vi "play_FXP_AFMss_MPC_DistEst_singleAxisN22.vi"() -> ()   [LabVIEW 2017]
uses:
  fpga_VIs/fixed-point/single-axis/fxp_mpc/fgm_pipiline/quadProgParams_pipe.ctl
  fpga_VIs/fixed-point/typeDefs/FXPControlParams_distEst.ctl
  <vilib>/Analysis/Matrix/Datatypes/RealMatrix.ctl
  fpga_fp_interface_lib/fpga_interface_types/boolean_indicators.ctl
  controls/ObserverMatrices.ctl
  <vilib>/userdefined/High Color/nirio_resource_hc.ctl
  <vilib>/Utility/error.llb/DialogType.ctl
  <vilib>/Utility/file.llb/Read Delimited Spreadsheet (DBL).vi
  <vilib>/FPGAPlugInAG/cRIO-9082/niLvFpga_Open_cRIO-9082.vi
  <vilib>/rvi/interface/common/dynamic/niFpgaDynamicAddResources.vi
  <vilib>/FPGAPlugInAG/Dynamic/niLvFpga_Reset_Dynamic.vi
  <vilib>/rvi/interface/common/niFpgaWaitOnOcc.vi
  <vilib>/Utility/error.llb/Error Cluster From Error Code.vi
  <vilib>/rvi/errors/niLvFpgaAdjustHostInterfaceError.vi
  <vilib>/FPGAPlugInAG/Dynamic/niLvFpga_Run_Dynamic.vi
  <vilib>/RVI Host/nirviSupport.llb/nirviErrorClusterFromErrorCode.vi
  fpga_fp_interface_lib/write_FP_data_to_fpga.vi
  fpga_fp_interface_lib/acquire_FXP_18-5_FIFO_1.vi
  <vilib>/Analysis/Matrix/Numeric/Conversions/Array To Matrix - RA2.vi
  <vilib>/Utility/file.llb/Write To Spreadsheet File (DBL).vi
  <vilib>/FPGAPlugInAG/Dynamic/niLvFpga_Close_Dynamic.vi
  <vilib>/rvi/interface/nirviOpenFPGA/nirviOpenFPGA.xnode
  FPGA Bitfiles/XYpeizocontrol_FPGATargetSPARTA_FXP_AFMss_MPC_singleAxis_N22.lvbitx
  <vilib>/rvi/interface/nirviMethod/nirviMethod.xnode
  <vilib>/rvi/interface/nirviReadWriteControl/nirviReadWriteControl.xnode
  <vilib>/rvi/interface/nirviCloseFPGA/nirviCloseFPGA.xnode
  <vilib>/rvi/errors/niLvFpgaMergeErrorWithErrorCode.vi
  <vilib>/rvi/interface/Simulation/niFpgaSimulationCallBeginRW.vi
  <vilib>/rvi/interface/nirviMethod/StockFPGA_InlinedMethodWaitForSingleIRQ.vi
  <vilib>/FPGAPlugInAG/Dynamic/niLvFpga_WaitOnIrq_Dynamic.vi
  <vilib>/FPGAPlugInAG/Dynamic/niLvFpga_AcknowledgeIrq_Dynamic.vi
  <vilib>/FPGAPlugInAG/Dynamic/niLvFpga_ConfigureFifo_Dynamic.vi
  NiFpgaLv.dll
  <vilib>/Analysis/Matrix/NI_Matrix.lvlib
  <vilib>/FPGAPlugInAG/Dynamic/niLvFpga_WriteFifo_Dynamic.vi
  labview/utils_lib/utils.lvlib
panel:
  out "size(s) 4":i32
  out "error out":errorcluster
  out "size(s) 3":i32
  out "size(s) 2":i32
  in  "N_sat":i32
  in  "sat_ws":T1
  in  "sat_ds":T1
  out "Actual Depth":u32
  out "first row":dbl[](array[numeric])
  out "elements left":i32=1
  in  "N_hyst":i32
  in  "w_s":T1
  in  "r_s":T1
  in  "TF Order":i32
  in  "den":T1
  in  "num":T1
  out "u_k out":fxp<+/-,32,5>
  out "size(s)":i32[](array[numeric])
  in  "Tab Control":T2(tab)
  in  "traj_path":path=path "Z:/mpc-journal/step-exps/traj_data.csvtraj_data.csv"
  in  "control_data_path":path=path "Z:/mpc-journal/step-exps/MPCControls01.csv"
  in  "outputDataPath":path=path "Z:/mpc-journal/step-exps/expOut_multiAxis_mpc_tmp.csv"
  in  "dry_run":bool
  out "XY Graph":cluster{dbl[], "2D Data Out":dbl[]}[](graph)
  out "QP_params":T3={"maxIter"=0, "nuN"=24, "Ns_mpc"=0, "-beta"=-0.9987945556640625, "beta+1"=1.9987945556640625}
  out "ControlParams":T4={"umax"=3.0, "Ns_obs/cntrl"=0, "ref_f_VEC"=[0.0, 0.0], "du_max"=0.0}
  in  "TsTicks":i32=1600
  in  "umax":dbl=1.0 format="%#_13g"
  in  "ymax":dbl=4.0 format="%#_13g"
  in  "Iters":i32=25
  in  "SettleTicks":i32=10
  in  "ABORT":bool
  out "Fifo matrix TimeOUt":bool
  in  "ref":dbl=1.0 format="%#_13g"
  out "Loop Ticks (benchmark)":i16
  in  "maxIter":u16=22
  in  "du_max":dbl=1.0 format="%#_13g"
  out "boolean  indicators":T5
  out "error out (stage 2)":errorcluster
  out "Error Out (stage 1)":errorcluster
  out "x-x(0)":fxp<+/-,18,5>
  out "ControlMatrices":T6
  out "MPC matrices":dbl[][](array[numeric])
  out "result_data":T1
  out "Empty Elements Remaining":u32
  # "NOTE: Ns is the number of states in the plant. The number of states in the \nobserver is Ns+1. Thus, for B, L, C, and A, we use NS+1. For K and Xss, we use Ns\nbecause the controller does not operate on the disturbance state, Xd."
  # "yk\nulin\ndu\nu_inv\nIpow\nX"
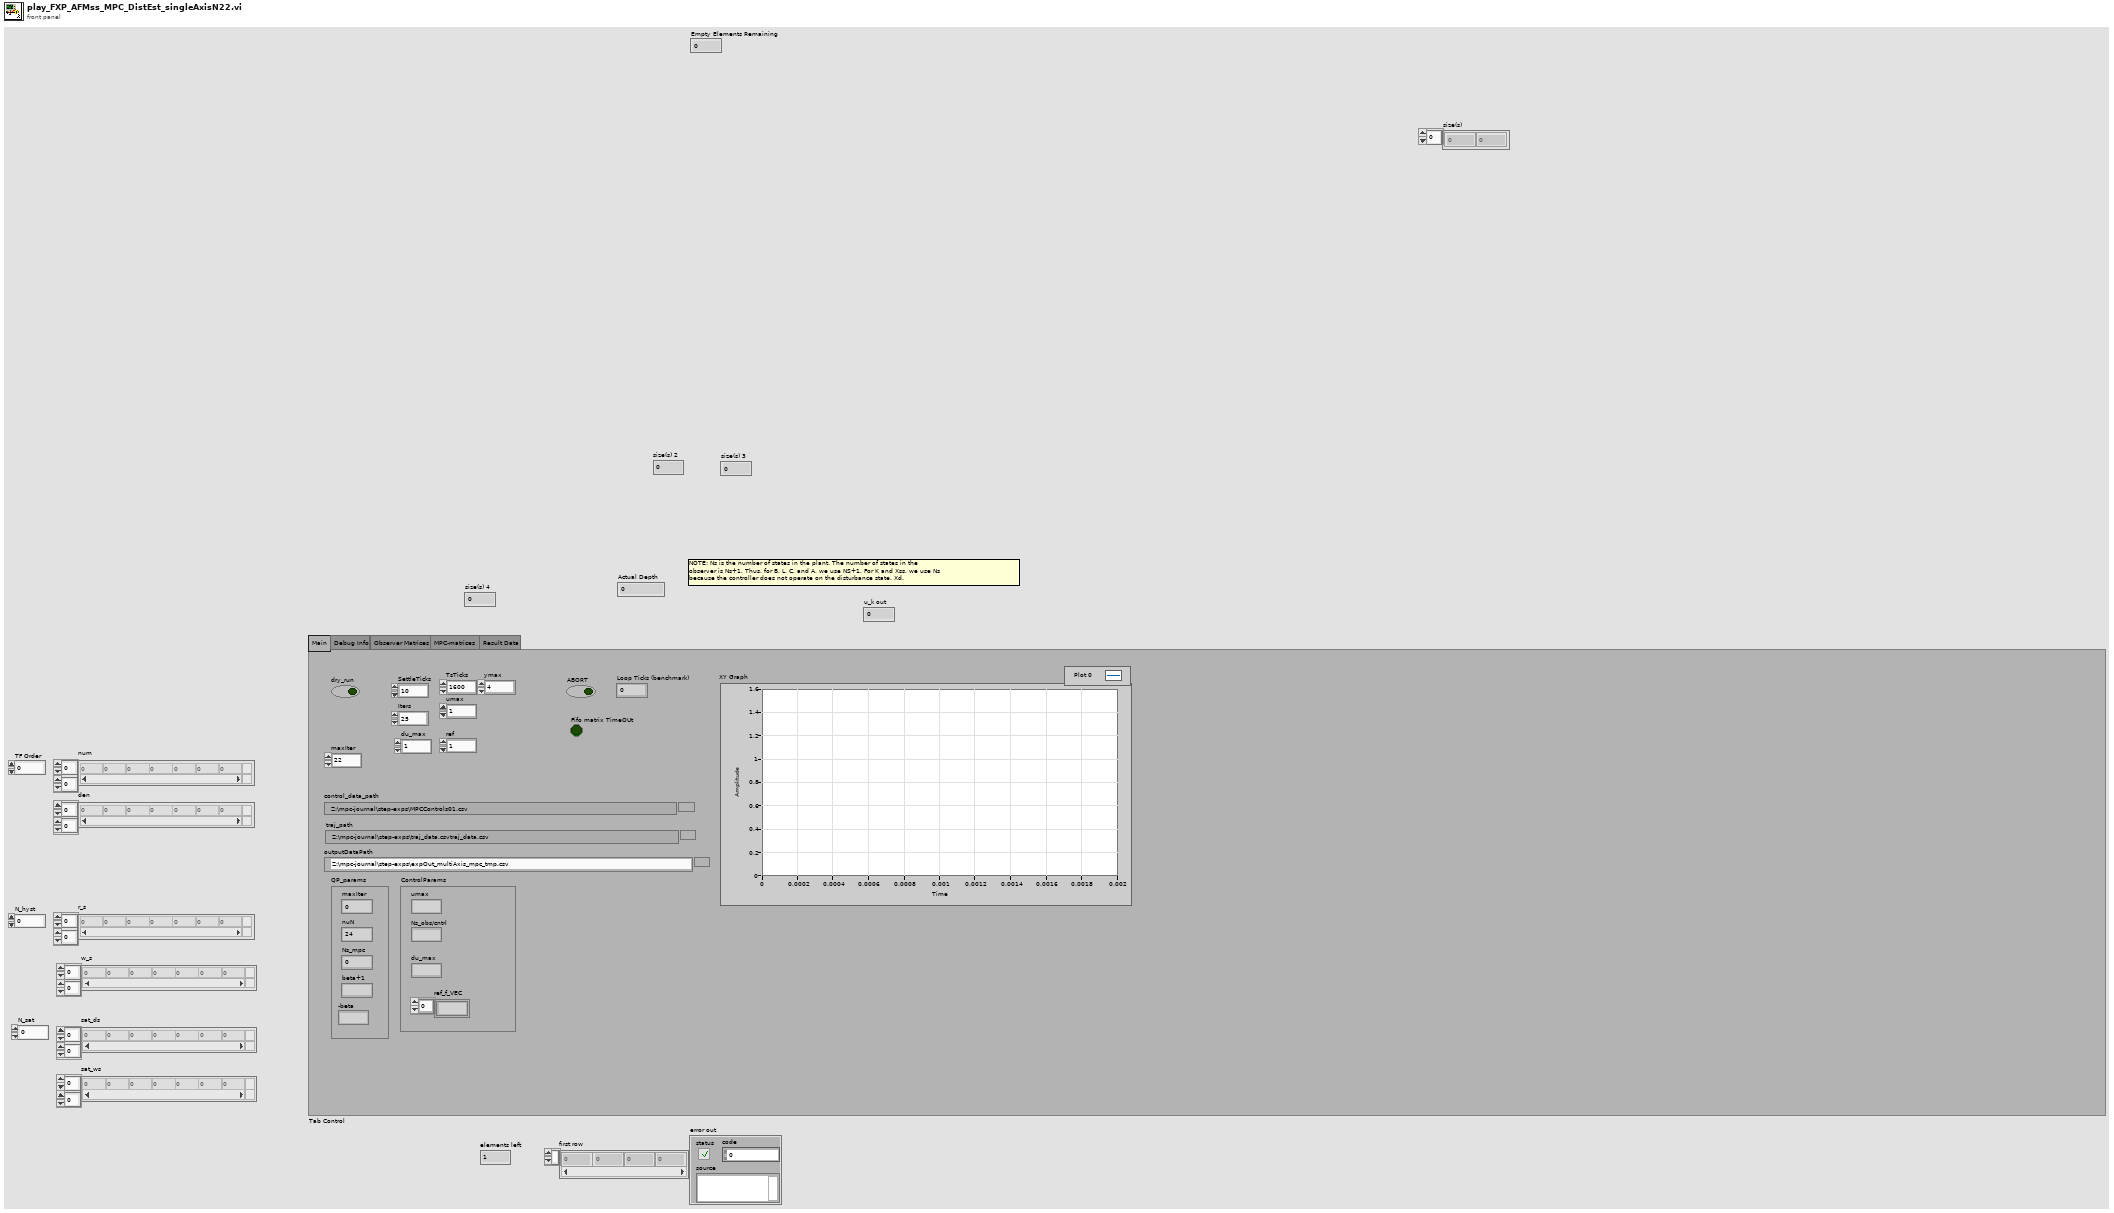
[diagram p1: front panel]
types:
  T1 = typedef "NI_Matrix.lvlib/RealMatrix.ctl" = dbl[][]
  T2 = enum32{"Main", "Debug Info", "Observer Matrices", "MPC-matrices", "Result Data"}
  T3 = typedef "quadProgParams_pipe.ctl" = cluster{"maxIter":u16, "nuN":u16, "Ns_mpc":u16, "-beta":fxp<+/-,18,2>, "beta+1":fxp<+/-,18,2>}
  T4 = typedef "FXPControlParams_distEst.ctl" = cluster{"umax":fxp<+/-,18,5>, "Ns_obs/cntrl":u8, "ref_f_VEC":fxp<+/-,32,5>[], "du_max":fxp<+/-,18,5>}
  T5 = typedef "boolean_indicators.ctl" = cluster{"unstable-z-traj":bool, "input fifo time-out":bool, "logging fifo timeout":bool, "scanning finished":bool, "unstable-x-traj":bool, "unstable-y-traj":bool, "ABORT":bool, "All Measurements Done":bool, "fpga_finished":bool}
  T6 = typedef "ObserverMatrices.ctl" = cluster{"Az":fxp<+/-,32,4>[][], "Bz":dbl[][], "Lz":dbl[][], "Kz":dbl[][], "NxNu":dbl[][]}
  T7 = typedef "nirio_resource_hc.ctl" = tag
  T8 = cluster{"unstable-z-traj":bool, "input fifo time-out":bool, "logging fifo timeout":bool, "scanning finished":bool, "unstable-x-traj":bool, "unstable-y-traj":bool, "ABORT":bool, "All Measurements Done":bool, "fpga_finished":bool}
  T9 = typedef "DialogType.ctl" = u16
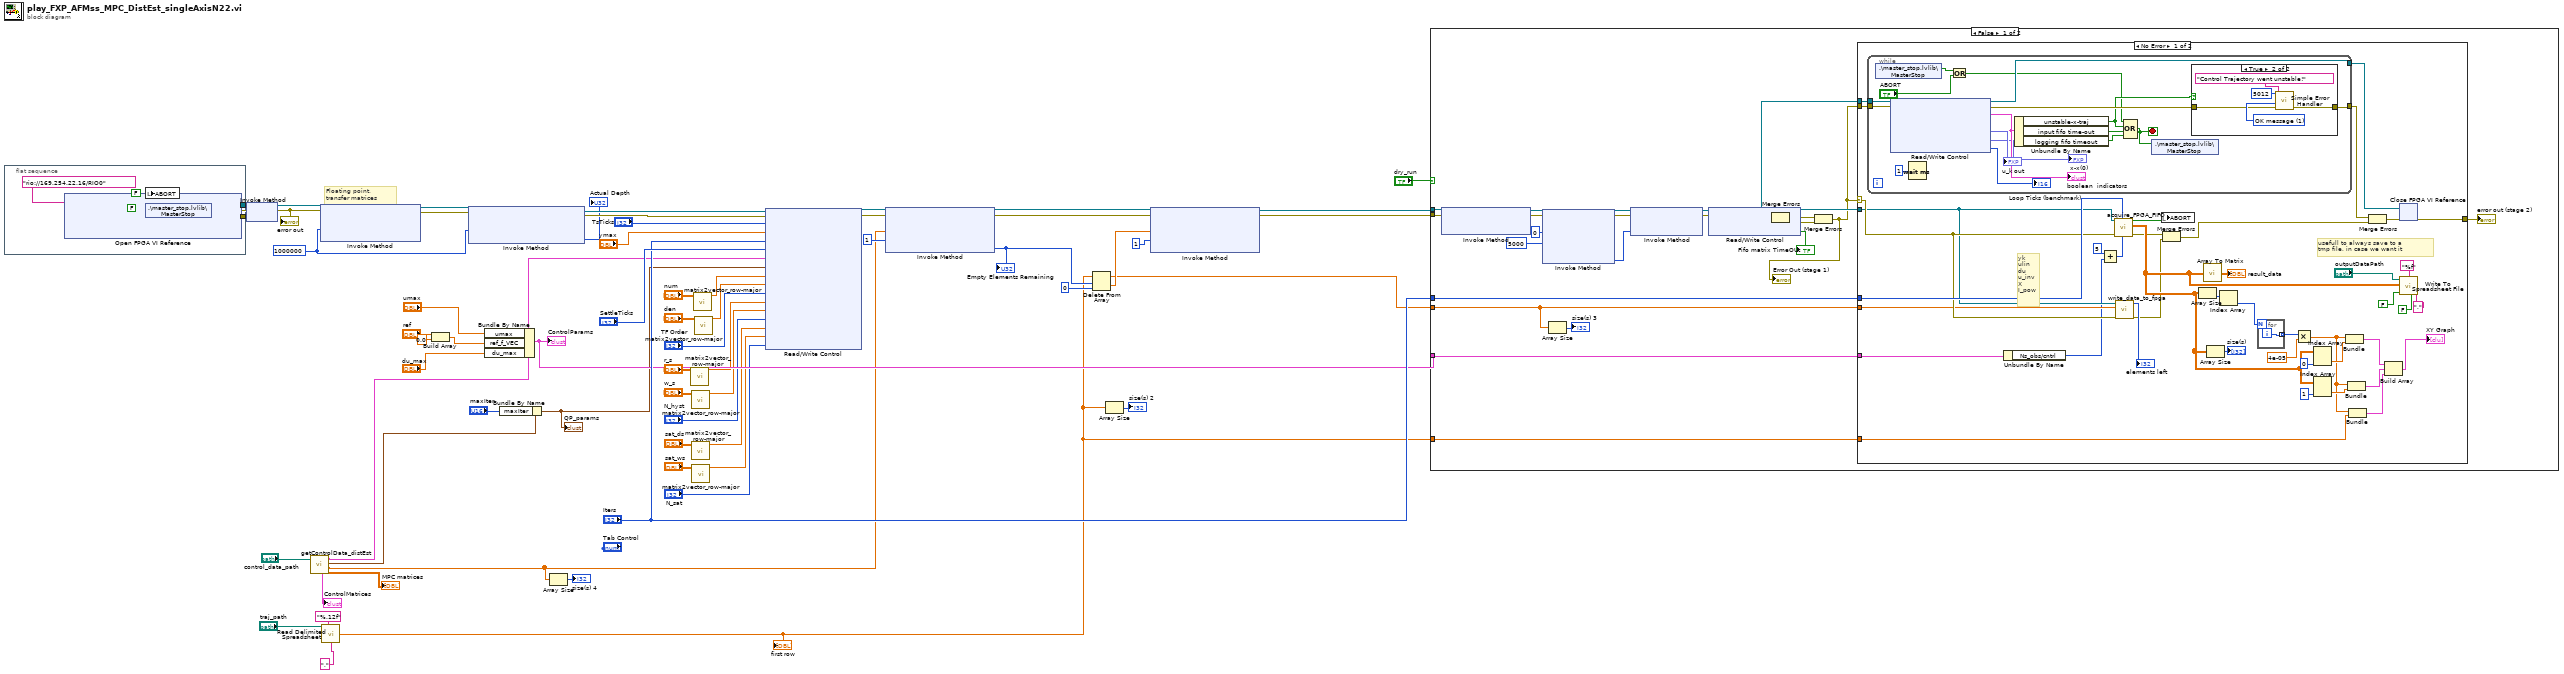
[diagram p0: block diagram]
diagram:
  w43 = u32 1000000 ("Requested Depth")
  # "Floating point, \ntransfer matrices"
  n1 = flat-sequence {
    tunnel: [w65] -> w56
    tunnel: [w67] -> w54
    frame #0 {
      n2 = xnode "Open FPGA VI Reference"("resource name"=T7 "rio://169.254.22.16/RIO0") -> ("FPGA VI Reference Out"=w67:refnum<k20>, "error out"=w64:errorcluster)  [unwired: 1 in]
      n3 = shared-variable ".\\master_stop.lvlib\\MasterStop"(FALSE ("MasterStop"), error in=w64) -> (error out=w65:errorcluster)
      n4 = local write "ABORT"(FALSE ("ABORT")) -> ()
    }
  }
  n5 = xnode "Invoke Method"("FPGA VI Reference In"=w54, "error in"=w56) -> ("FPGA VI Reference Out"=w53:refnum<k20>, "error out"=w52:errorcluster)
  "error out" <- w52
  n6 = call "getControlData_distEst.vi"("system matricec path"="control_data_path") -> ("MPC matrices"=→"MPC matrices":dbl[][], "AllMatrix"=w2:dbl[], "QP_params"=w36:T3, "ControlParams"=w41:T4, "ControlMatrices"=→"ControlMatrices":T6)  [unwired: 6 in]
  n7 = xnode "Invoke Method"("FPGA VI Reference In"=w53, "error in"=w52, "Requested Depth"=w43) -> ("FPGA VI Reference Out"=w51:refnum<k20>, "error out"=w50:errorcluster)  [unwired: 1 out]
  n8 = call-poly <vilib>:"Read Delimited Spreadsheet.vi"("file path (dialog if empty)"="traj_path", "format (%.3f)"="%.12f", "delimiter (\\t)"="," ("format (%.3f)")) -> ("first row"=w4:dbl[])  [unwired: 7 in, 5 out]
  "first row" <- w4
  n9 = Build Array("ref", 0.0 ("element")) -> (w37:dbl[])
  n10 = xnode "Invoke Method"("FPGA VI Reference In"=w51, "error in"=w50, "Requested Depth"=w43) -> ("FPGA VI Reference Out"=w49:refnum<k20>, "error out"=w48:errorcluster, "Actual Depth"=→"Actual Depth":u32)
  n11 = Bundle By Name(cluster=w41, "umax"="umax", "ref_f_VEC"=w37, "du_max"="du_max") -> (w40:T4)
  "ControlParams" <- w40
  n12 = Bundle By Name(cluster=w36, "maxIter"="maxIter") -> (w34:T3)
  "QP_params" <- w34
  n13 = Array Size(array=w2) -> (size(s)=→"size(s) 4":i32)
  n14 = call "matrix2vector_row-major.vi"("Matrix"="r_s") -> ("vector"=w26:dbl[])  [unwired: 10 in]
  n15 = call "matrix2vector_row-major.vi"("Matrix"="w_s") -> ("vector"=w25:dbl[])  [unwired: 10 in]
  n16 = call "matrix2vector_row-major.vi"("Matrix"="sat_ds") -> ("vector"=w8:dbl[])  [unwired: 10 in]
  n17 = call "matrix2vector_row-major.vi"("Matrix"="sat_ws") -> ("vector"=w7:dbl[])  [unwired: 10 in]
  n18 = call "matrix2vector_row-major.vi"("Matrix"="num") -> ("vector"=w29:dbl[])  [unwired: 10 in]
  n19 = call "matrix2vector_row-major.vi"("Matrix"="den") -> ("vector"=w28:dbl[])  [unwired: 10 in]
  n20 = xnode "Read/Write Control"("FPGA VI Reference In"=w49, "error in"=w48, "TsTicks"="TsTicks", "ymax"="ymax", "iters"="Iters", "Settle Ticks"="SettleTicks", "ControlParams_distEst"=w40, "QP_params"=w34, "Num"=w29, "Den"=w28, "TF Order"="TF Order", "r_s"=w26, "w_s"=w25, "N_hyst"="N_hyst", "sat_d_s"=w8, "sat_w_s"=w7, "N_sat"="N_sat") -> ("FPGA VI Reference Out"=w59:refnum<k20>, "error out"=w58:errorcluster)
  n21 = xnode "Invoke Method"("FPGA VI Reference In"=w59, "error in"=w58, "Data"=w2, "Timeout (ms)"=1) -> ("FPGA VI Reference Out"=w20:refnum<k20>, "error out"=w19:errorcluster, "Empty Elements Remaining"=w15:u32)
  "Empty Elements Remaining" <- w15
  n22 = Delete From Array(array=w4, length=w15, index=0) -> (deleted portion=w14:dbl[], array with subset deleted=w12:dbl[])
  n23 = Array Size(array=w4) -> (size(s)=→"size(s) 2":i32)
  n24 = xnode "Invoke Method"("FPGA VI Reference In"=w20, "error in"=w19, "Data"=w14, "Timeout (ms)"=1) -> ("FPGA VI Reference Out"=w18:refnum<k20>, "error out"=w17:errorcluster)  [unwired: 1 out]
  n25 = case shown="False" "dry_run" {
    tunnel: w17 -> [w91 _]
    tunnel: "Iters" -> [w79 _]
    tunnel: w40 -> [w77 _]
    tunnel: w18 -> [w72 _]
    tunnel: w12 -> [w69 _]
    tunnel: w4 -> [w71 _]
    frame False {
      n26 = xnode "Invoke Method"("FPGA VI Reference In"=w72, "error in"=w91) -> ("FPGA VI Reference Out"=w82:refnum<k20>, "error out"=w83:errorcluster)  [unwired: 1 in]
      n27 = xnode "Invoke Method"("FPGA VI Reference In"=w82, "error in"=w83, "IRQ Number(s)"=0, "Timeout (ms)"=5000) -> ("FPGA VI Reference Out"=w88:refnum<k20>, "error out"=w89:errorcluster, "IRQ(s) Asserted"=w85:i32)  [unwired: 1 out]
      n28 = Array Size(array=w69) -> (size(s)=→"size(s) 3":i32)
      n29 = xnode "Invoke Method"("FPGA VI Reference In"=w88, "error in"=w89, "IRQ Number(s)"=w85) -> ("FPGA VI Reference Out"=w87:refnum<k20>, "error out"=w86:errorcluster)
      n30 = xnode "Read/Write Control"("FPGA VI Reference In"=w87, "error in"=w86) -> ("FPGA VI Reference Out"=w78:refnum<k20>, "error out"=w90:errorcluster, "Error Out"=w74:errorcluster, "Matrix FIFO  TimeOut"=→"Fifo matrix TimeOUt":bool)
      n31 = Merge Errors(w90, w74) -> (w75:errorcluster)
      n32 = Merge Errors(w75, w74) -> (w73:errorcluster)
      "Error Out (stage 1)" <- w73
      n33 = case shown="No Error" w73 {
        selector: w73 -> [w107 w157]
        tunnel: [w131 w157] -> w80
        tunnel: w78 -> [w130 _]
        tunnel: w73 -> [w129 _]
        tunnel: w79 -> [w126 _]
        tunnel: w78 -> [w106 _]
        tunnel: w77 -> [w93 _]
        tunnel: w71 -> [w100 _]
        tunnel: w69 -> [w98 _]
        frame No Error {
          # "yk\nulin\ndu\nu_inv\nX\nI_pow"
          # "usefull to always save to a \ntmp file, in case we want it"
          n34 = while {
            tunnel: w130 -> [w149]
            tunnel: w129 -> [w148]
            tunnel: [w146] -> w128
            tunnel: [w145] -> w127
            stop <- w144 stop-if-true
            n35 = shared-variable ".\\master_stop.lvlib\\MasterStop"() -> (w139:bool)  [unwired: 1 in, 1 out]
            n36 = xnode "Read/Write Control"("FPGA VI Reference In"=w149, "error in"=w148) -> ("FPGA VI Reference Out"=w145:refnum<k20>, "error out"=w147:errorcluster, "boolean  indicators"=w143:T8, "x-x(0)"=→"x-x(0)":fxp<+/-,18,5>, "u_k"=→"u_k out":fxp<+/-,32,5>, "Loop Ticks (benchmark)"=→"Loop Ticks (benchmark)":i16)  [unwired: 1 out]
            "boolean  indicators" <- w143
            n37 = Wait (ms)(milliseconds to wait=u32 1) -> ()  [unwired: 1 out]
            n38 = Or(x=w139, y="ABORT") -> (x .or. y?=w137:bool)
            n39 = Unbundle By Name(w143) -> ("unstable-x-traj"=w141:bool, "input fifo time-out"=w142:bool, "logging fifo timeout"=w140:bool)
            n40 = Compound Arithmetic op=OR(w137, w141, w142, w140) -> (w144:bool)
            n41 = shared-variable ".\\master_stop.lvlib\\MasterStop"(w144) -> ()  [unwired: 1 in, 1 out]
            n42 = case shown="True" w141 {
              tunnel: w147 -> [w151 w153]
              tunnel: [w151 w152] -> w146
              frame False {
              }
              frame True {
                w156 = T9 1 items=["no dialog", "OK message", "continue or stop message", "OK message + warnings", "continue/stop + warnings"] ("type of dialog (OK msg:1)")
                n43 = call <vilib>:"Simple Error Handler.vi"("error code (no error:0)"=5012, "error source (\" \")"="Control Trajectory went unstable!" ("error source (\" \")"), "type of dialog (OK msg:1)"=w156, "error in (no error)"=w153) -> ("error out"=w152:errorcluster)  [unwired: 1 in, 4 out]
              }
            }
          }
          n44 = Unbundle By Name(w93) -> ("Ns_obs/cntrl"=w92:u8)
          n45 = Add(x=u8 5 ("y"), y=w92) -> (x+y=w94:u8)
          n46 = call-poly "acquire_FPGA_FIFO.vi"("numChannels"=w94, "Iters"=w126, "error in"=w107, "FPGA Interface"=w106) -> ("error out"=w104:errorcluster, "2D Data Out"=w108:dbl[][], "acquisition done"=w125:bool)  [unwired: 3 in, 2 out]
          n47 = call-poly "write_data_to_fpga.vi"("error in"=w107, "all rows"=w98, "FPGA Interface"=w106) -> ("error out"=w102:errorcluster, "elements left"=→"elements left":i32)  [unwired: 7 in]
          n48 = local write "ABORT"(w125) -> ()
          n49 = Merge Errors(w104, w102) -> (w103:errorcluster)
          n50 = Array Size(array=w108) -> (size(s)=w120:i32[])
          n51 = call-poly <vilib>:"Array To Matrix.vi"("Real 2D Array"=w108) -> ("Real Matrix"=→"result_data":T1)
          n52 = Array Size(array=w108) -> (size(s)=→"size(s)":i32[])
          n53 = Index Array(array=w120) -> (element=w119:i32)  [unwired: 1 in]
          n54 = for {
            N: w119 -> [_]
            tunnel: [w133] -> w118 mode=indexing
            i -> [w133]
          }
          n55 = Multiply(x=w118, y=4e-05) -> (x*y=w101:dbl[])
          n56 = Index Array(array=w108, index (col)=0 ("disabled index (col)")) -> (element=w116:dbl[])  [unwired: 1 in]
          n57 = Index Array(array=w108, index (col)=1 ("index (row)")) -> (element=w115:dbl[])  [unwired: 1 in]
          n58 = Bundle(w101, "2D Data Out"=w116) -> (w113:cluster{dbl[], "2D Data Out":dbl[]})  [unwired: 1 in]
          n59 = Bundle(w101, "2D Data Out"=w115) -> (w114:cluster{dbl[], "2D Data Out":dbl[]})  [unwired: 1 in]
          n60 = Bundle(w101, "first row"=w100) -> (w99:cluster{dbl[], "first row":dbl[]})  [unwired: 1 in]
          n61 = Merge Errors(w128, w103) -> (w132:errorcluster)
          n62 = Build Array(w113, w114, w99) -> (→"XY Graph":cluster{dbl[], "first row":dbl[]}[])
          n63 = xnode "Close FPGA VI Reference"("FPGA VI Reference In"=w127, "error in"=w132) -> ("error out"=w131:errorcluster)
          n64 = call-poly <vilib>:"Write To Spreadsheet File.vi"("delimiter (\\t)"=",", "transpose? (no:F)"=FALSE, "format (%.3f)"="%f", "append to file? (new file:F)"=FALSE, "2D data"=w108, "file path (dialog if empty)"="outputDataPath") -> ()  [unwired: 2 in, 1 out]
        }
        frame Error {
        }
      }
      "error out (stage 2)" <- w80
    }
    frame True {
    }
  }
